vi "Dye Whole Recipe Table.vi"(8 "error in (no error)":errorcluster, 11 "Kitchen Actor in":refnum<class "Kitchen Actor.lvclass">) -> (0 "error out":errorcluster, 3 "Kitchen Actor out":refnum<class "Kitchen Actor.lvclass">)   [LabVIEW 2024, in "Kitchen Actor.lvlib" / "Kitchen Actor.lvclass"]
uses:
  Kitchen Actor.lvclass
  Kitchen Actor.lvclass/Kitchen Actor.ctl
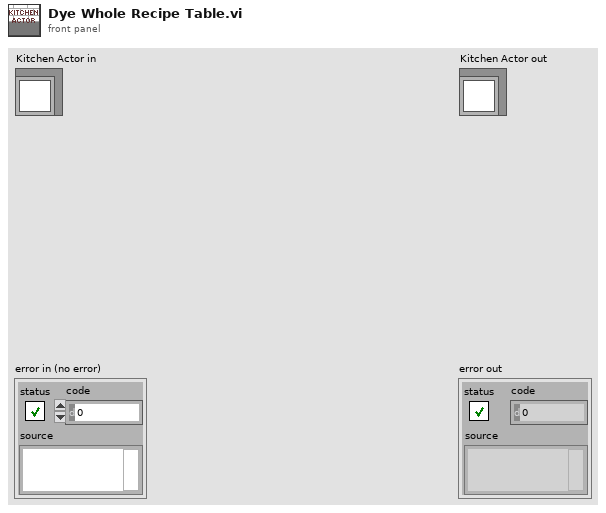
[diagram p1: front panel]
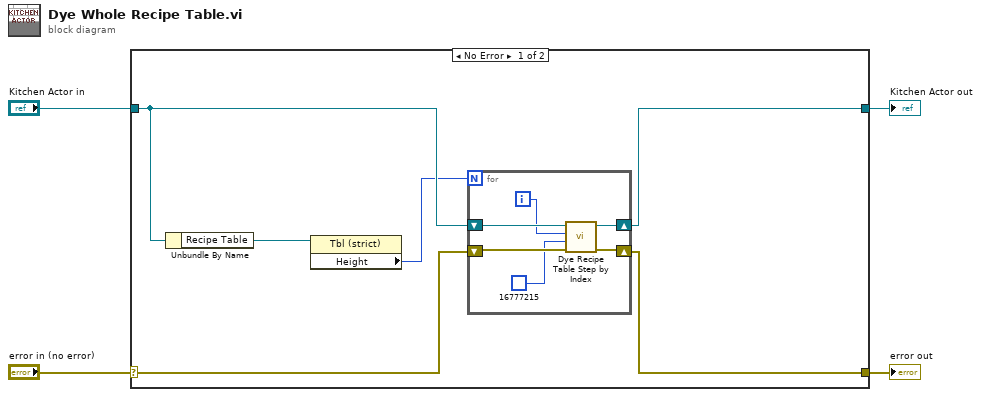
[diagram p0: block diagram]
diagram:
  n1 = case shown="No Error" "error in (no error)" {
    selector: "error in (no error)" -> [w9 w18]
    tunnel: [w8 w18] -> w3
    tunnel: [w10 w17] -> w1
    tunnel: "Kitchen Actor in" -> [w7 w17]
    frame No Error {
      n2 = Unbundle By Name(w7) -> ("Recipe Table"=w6:refnum<vi>)
      n3 = property class="Tbl (strict)"(reference=w6) -> ("Height"=w5:u32)  [unwired: 1 in, 2 out]
      n4 = for {
        N: w5 -> [_]
        shift-right: [w15] -> w10
        shift-left: w7 -> [w16]
        shift-right: [w13] -> w8
        shift-left: w9 -> [w14]
        i -> [w12]
        n5 = call-dynamic "Dye Recipe Table Step by Index.vi"("error in (no error)"=w14, "Dye Color"=u32 16777215, "Index"=w12, "Kitchen Actor in"=w16) -> ("error out"=w13:errorcluster, "Kitchen Actor out"=w15:refnum<class "Kitchen Actor.lvclass">)  [unwired: 6 in]
      }
    }
    frame Error {
    }
  }
  "error out" <- w3
  "Kitchen Actor out" <- w1
